vi "Set Sweep Dwell.vi"(8 "error in (no error)":errorcluster, 10 "Sweep Dwell Time":dbl[unit], 11 "VISA resource name":refnum<visa-resource-name>) -> (0 "error out":errorcluster, 3 "VISA resource name out":refnum<visa-resource-name>)   [LabVIEW 2017, in "Agilent PSG MXG Series.lvlib"]
uses:
  Agilent PSG MXG Series.lvlib
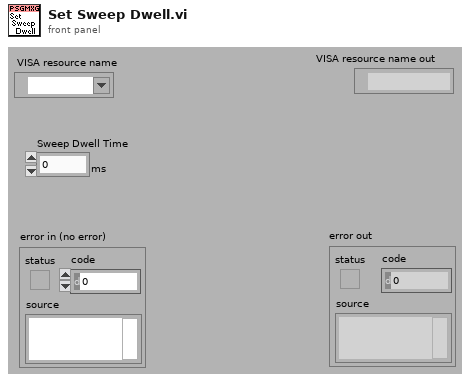
[diagram p1: front panel]
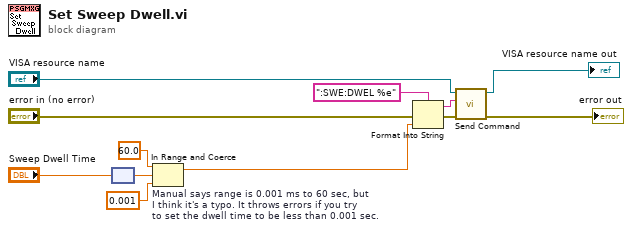
[diagram p0: block diagram]
diagram:
  n1 = node("Sweep Dwell Time") -> (w2:dbl)
  n2 = In Range and Coerce "Manual says range is 0.001 ms to 60 sec, but\nI think it's a typo. It throws errors if you try \nto set the dwell time to be less than 0.001 sec."(upper limit=60.0, x=w2, lower limit=0.001) -> (coerced(x)=w1:dbl)  [unwired: 1 out]
  n3 = Format Into String(format string=":SWE:DWEL %e", error in="error in (no error)", w1) -> (resulting string=w6:string, error out=w7:errorcluster)  [unwired: 1 in]
  n4 = call "Send Command.vi"("error in (no error)"=w7, "write buffer"=w6, "VISA resource name"="VISA resource name") -> ("error out"=→"error out":errorcluster, "VISA resource name out"=→"VISA resource name out":refnum<visa-resource-name>)  [unwired: 7 out]
